vi "Configure.vi"(8 "error in (no error)":errorcluster, 9 "Record":bool=TRUE, 10 "Recording Channels":refnum<k21>="All4498", 11 "IntanElectrophysiology in":refnum<class "IntanElectrophysiology.lvclass">) -> (0 "error out":errorcluster, 3 "IntanElectrophysiology out":refnum<class "IntanElectrophysiology.lvclass">)   [LabVIEW 2012, in "IntanElectrophysiology.lvclass"]
uses:
  IntanElectrophysiology.lvclass
  <vilib>/sound2/lvsound2.llb/Sampling Mode.ctl
  <vilib>/sound2/lvsound2.llb/Sound Data Format.ctl
  <resource>/objmgr/daqmx.rc
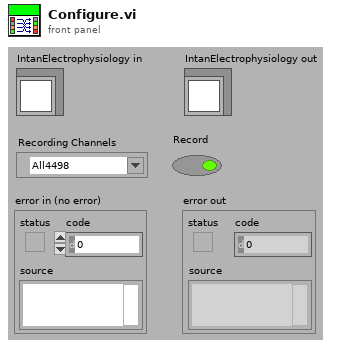
[diagram p1: front panel]
types:
  T1 = typedef "Sound Data Format.ctl" = cluster{"sample rate (S/s)":dbl, "number of channels":i32, "bits per sample":i32}
  T2 = typedef "Sampling Mode.ctl" = i32
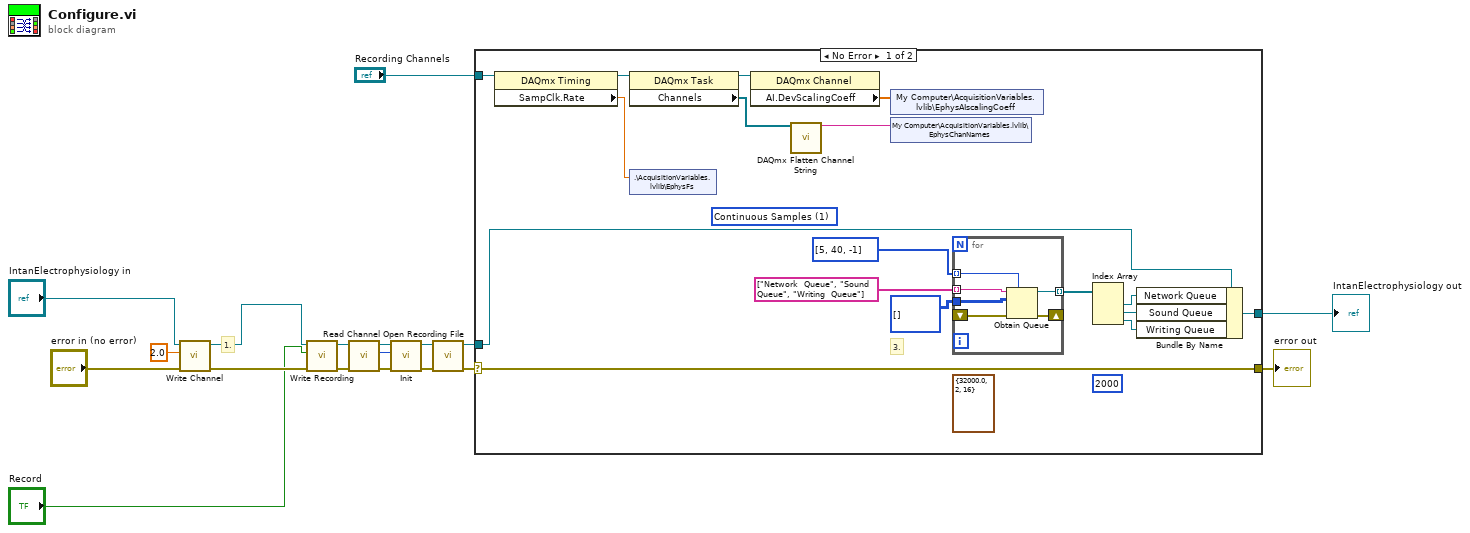
[diagram p0: block diagram]
diagram:
  # "1."
  n1 = call-dynamic "Write Channel.vi"("error in (no error)"="error in (no error)", "Channel"=2.0, "AcquistionObject in"="IntanElectrophysiology in") -> ("error out"=w6:errorcluster, "AcquistionObject out"=w7:refnum<class "IntanElectrophysiology.lvclass">)  [unwired: 7 in]
  n2 = call-dynamic "Write Recording.vi"("error in (no error)"=w6, "Recording"="Record", "AcquireTraces in"=w7) -> ("error out"=w3:errorcluster, "AcquireTraces out"=w8:refnum<class "IntanElectrophysiology.lvclass">)  [unwired: 7 in]
  n3 = call-dynamic "Read Channel.vi"("error in (no error)"=w3, "AcquistionObject in"=w8) -> ("error out"=w10:errorcluster, "Channel"=w12:i16, "AcquistionObject out"=w11:refnum<class "IntanElectrophysiology.lvclass">)  [unwired: 7 in]
  n4 = call-dynamic "Init.vi"("error in (no error)"=w10, "Channel"=w12, "AcquistionObject in"=w11) -> ("error out"=w9:errorcluster, "AcquistionObject out"=w1:refnum<class "IntanElectrophysiology.lvclass">)  [unwired: 7 in]
  n5 = call-dynamic "Open Recording File.vi"("error in (no error)"=w9, "IntanElectrophysiology in"=w1) -> ("error out"=w4:errorcluster, "IntanElectrophysiology out"=w5:refnum<class "IntanElectrophysiology.lvclass">)  [unwired: 8 in]
  n6 = case shown="No Error" w4 {
    selector: w4 -> [w20 w43]
    tunnel: [w20 w43] -> w14
    tunnel: [w29 w42] -> w13
    tunnel: w5 -> [w19 w42]
    tunnel: "Recording Channels" -> [w28 _]
    frame No Error {
      (unwired) T1 {"sample rate (S/s)"=32000.0, "number of channels"=2, "bits per sample"=16} ("sound format")
      (unwired) 2000 ("number of samples/ch")
      (unwired) T2 1 items=["Finite Samples", "Continuous Samples"] ("sample mode")
      # "3."
      n7 = property class="DAQmx Timing"(reference=w28) -> (reference out=w27:refnum<k21>, "SampClk.Rate"=w26:dbl)  [unwired: 1 in, 1 out]
      n8 = property class="DAQmx Task"(reference=w27) -> (reference out=w23:refnum<k21>, "Channels"=w25:refnum<k21>[])  [unwired: 1 in, 1 out]
      n9 = shared-variable ".\\AcquisitionVariables.lvlib\\EphysFs"(w26) -> ()  [unwired: 1 in, 1 out]
      n10 = property class="DAQmx Channel"(reference=w23) -> ("AI.DevScalingCoeff"=w22:dbl[])  [unwired: 1 in, 2 out]
      n11 = call <vilib>:"DAQmx Flatten Channel String.vi"("names in"=w25) -> ("names out"=w24:string)  [unwired: 13 in, 1 out]
      n12 = shared-variable "My Computer\\AcquisitionVariables.lvlib\\EphysAIscalingCoeff"(w22) -> ()  [unwired: 1 in, 1 out]
      n13 = shared-variable "My Computer\\AcquisitionVariables.lvlib\\EphysChanNames"(w24) -> ()  [unwired: 1 in, 1 out]
      n14 = for {
        tunnel: string[] ["Network  Queue", "Sound  Queue", "Writing  Queue"] -> [w41] mode=indexing
        tunnel: i32[][] [] -> [w40]
        tunnel: [w39] -> w33 mode=indexing
        shift-right: [w38] -> _
        shift-left: _ -> [w37]
        tunnel: i32[] [5, 40, -1] -> [w36] mode=indexing
        n15 = Obtain Queue(max queue size (-1, unlimited)=w36, name (unnamed)=w41, element data type=w40, error in (no error)=w37) -> (queue out=w39:refnum<queue>, error out=w38:errorcluster)  [unwired: 1 in, 1 out]
      }
      n16 = Index Array(array=w33) -> (element #1=w32:refnum<queue>, element #2=w31:refnum<queue>, element #3=w30:refnum<queue>)  [unwired: 3 in]
      n17 = Bundle By Name(cluster=w19, "Network Queue"=w32, "Sound Queue"=w31, "Writing Queue"=w30) -> (w29:refnum<class "IntanElectrophysiology.lvclass">)
    }
    frame Error {
    }
  }
  "error out" <- w14
  "IntanElectrophysiology out" <- w13
